vi "Translator.File.RemoveOldStrings.vi"(7 "group":string, 8 "error in":errorcluster, 9 "labels":string[](array[string]), 11 "refnum in":T1) -> (0 "error out":errorcluster, 1 "#removed":i32, 3 "refnum out":T1)   [LabVIEW 2016]
uses:
  <vilib>/Utility/config.llb/Config Data RefNum.ctl
  <vilib>/Utility/config.llb/NI_LVConfig.lvlib
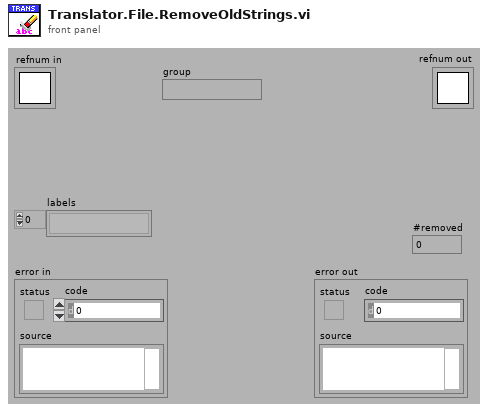
[diagram p1: front panel]
types:
  T1 = typedef "NI_LVConfig.lvlib/Config Data RefNum.ctl" = refnum<k1>
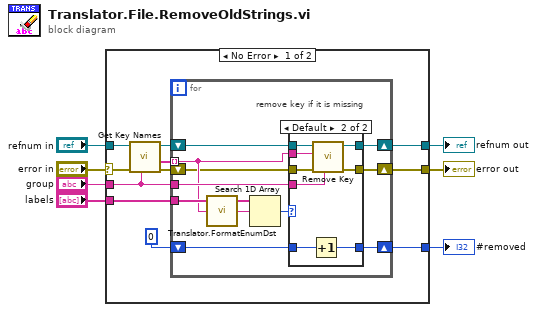
[diagram p0: block diagram]
diagram:
  n1 = case shown="No Error" "error in" {
    selector: "error in" -> [w10 w41]
    tunnel: [w18 _] -> w7
    tunnel: "refnum in" -> [w16 w42]
    tunnel: [w8 w42] -> w1
    tunnel: [w9 w41] -> w5
    tunnel: "group" -> [w12 _]
    tunnel: "labels" -> [w11 _]
    frame No Error {
      n2 = call <vilib>:"Get Key Names.vi"("section"=w12, "error in (no error)"=w10, "refnum"=w16) -> ("error out"=w15:errorcluster, "key names"=w13:string[], "refnum out"=w14:T1)  [unwired: 5 in, 1 out]
      n3 = for {
        shift-right: [w27] -> w9
        shift-left: w15 -> [w19]
        shift-right: [w29] -> w8
        shift-left: w14 -> [w28]
        tunnel: w13 -> [w20] mode=indexing
        tunnel: w11 -> [w22]
        tunnel: w12 -> [w25]
        shift-right: [w23] -> w18
        shift-left: 0 -> [w24]
        # "remove key if it is missing"
        n4 = call "Translator.FormatEnumDst.vi"("text in"=w20) -> ("text out"=w21:string)
        n5 = Search 1D Array(1D array=w22, element=w21) -> (index of element=w26:i32)  [unwired: 1 in]
        n6 = case shown="Default" w26 {
          tunnel: w19 -> [w32 w40]
          tunnel: [w31 w39] -> w29
          tunnel: w28 -> [w31 w38]
          tunnel: w20 -> [_ w37]
          tunnel: [w32 w36] -> w27
          tunnel: w25 -> [_ w33]
          tunnel: w24 -> [w30 w35]
          tunnel: [w30 w34] -> w23
          frame 0.. {
          }
          frame Default {
            n7 = Increment(x=w35) -> (x+1=w34:i32)
            n8 = call <vilib>:"Remove Key.vi"("section"=w33, "error in (no error)"=w40, "key"=w37, "refnum"=w38) -> ("error out"=w36:errorcluster, "refnum out"=w39:T1)  [unwired: 5 in, 1 out]
          }
        }
      }
    }
    frame Error {
    }
  }
  "#removed" <- w7
  "refnum out" <- w1
  "error out" <- w5
